vi "NumericPad-DM.vi"(0 "Input Cluster":T2={"Operation"=0, "Wait for (ms):"=1000, "Look for key press:"=49} {"Look for key press:" items=["Key_1"=49, "Key_2"=50, "Key_3"=51, "Key_4"=52, "Key_5"=53, "Key_6"=54, "Key_7"=55, "Key_8"=56, "Key_9"=57, "Key_0"=48, "Key_#"=35, "Key_*"=42]; "Operation" items=["ReadPad", "InitializeSetup"]}, 2 "NXT":T3={"error"={"status"=FALSE, "code"=0, "source"=""}, "address"="USB0::0x0694::0x0002::001653FF017B::RAW", "NXT #"=0, "Show Error"=TRUE, "Connection"=4} {"Connection" items=["USB", "Bluetooth", "USB then Bluetooth", "Last Connection", "Preference"]}, 3 "Input Port":T4 items=["Port 1", "Port 2", "Port 3", "Port 4"]) -> (1 "Output Cluster":T1={"Key Numeric Value"=49, "Key String Value"="1", "Key match found"=FALSE}, 4 "NXT dup":T3={"error"={"status"=FALSE, "code"=0, "source"=""}, "address"="USB0::0x0694::0x0002::001653FF017B::RAW", "NXT #"=0, "Show Error"=TRUE, "Connection"=4} {"Connection" items=["USB", "Bluetooth", "USB then Bluetooth", "Last Connection", "Preference"]})   [LabVIEW 2009]
uses:
  <vilib>/NXT/Subs/LVHSConnector.ctl
  <vilib>/NXT/Block Support/NXT_InputPort.ctl
  <vilib>/NXT/Block Support/HWPage.SensorType.ctl
  <vilib>/NXT/Block Support/HWPage.SensorMode.ctl
  <vilib>/NXT/Dual Mode Library/Waits/Wait_Num(msec).vi
panel:
  out "Look for key press:":u8(ring)=49 caption="Operation" items=["Key_1"=49, "Key_2"=50, "Key_3"=51, "Key_4"=52, "Key_5"=53, "Key_6"=54, "Key_7"=55, "Key_8"=56, "Key_9"=57, "Key_0"=48, "Key_#"=35, "Key_*"=42]
  out "Key match found":bool
  in  "keymapS":string[](array[string])=[" ", " ", " ", " ", "4", "1", "7", "*", "5", "2", "8", "0", "3", "6", "9", "#"]
  out "Key String Value":string="1"
  in  "keyMapN":u8[](array[numeric])=[0, 0, 0, 0, 52, 49, 55, 42, 53, 50, 56, 48, 51, 54, 57, 35, 119] format="%x"
  out "Key Numeric Value":u8=49
  out "KeyPos":u8=5 format="%x"
  # "mindsensors.com\nCopyright (c) 2009 by mindsensors.com\nEmail: info (<at>) mindsensors (<dot>) com\n\nThis program is free software. You can redistribute it and/or modify\nit under the terms of the GNU General Public License as published by\nthe Free Software Foundation; version 3 of the License.\nRead the license at: http://www.gnu.org/licenses/gpl.txt"
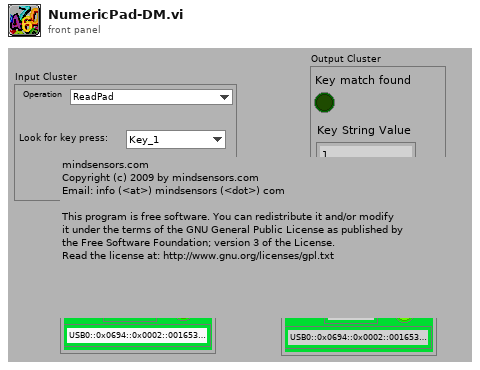
[diagram p1: front panel]
types:
  T1 = cluster{"Key Numeric Value":u8, "Key String Value":string, "Key match found":bool}
  T2 = cluster{"Operation":u8, "Wait for (ms):":i16, "Look for key press:":u8}
  T3 = typedef "LVHSConnector.ctl" = cluster{"error":errorcluster, "address":string, "NXT #":i32, "Show Error":bool, "Connection":u16}
  T4 = typedef "NXT_InputPort.ctl" = u8
  T5 = typedef "HWPage.SensorType.ctl" = u8
  T6 = typedef "HWPage.SensorMode.ctl" = u8
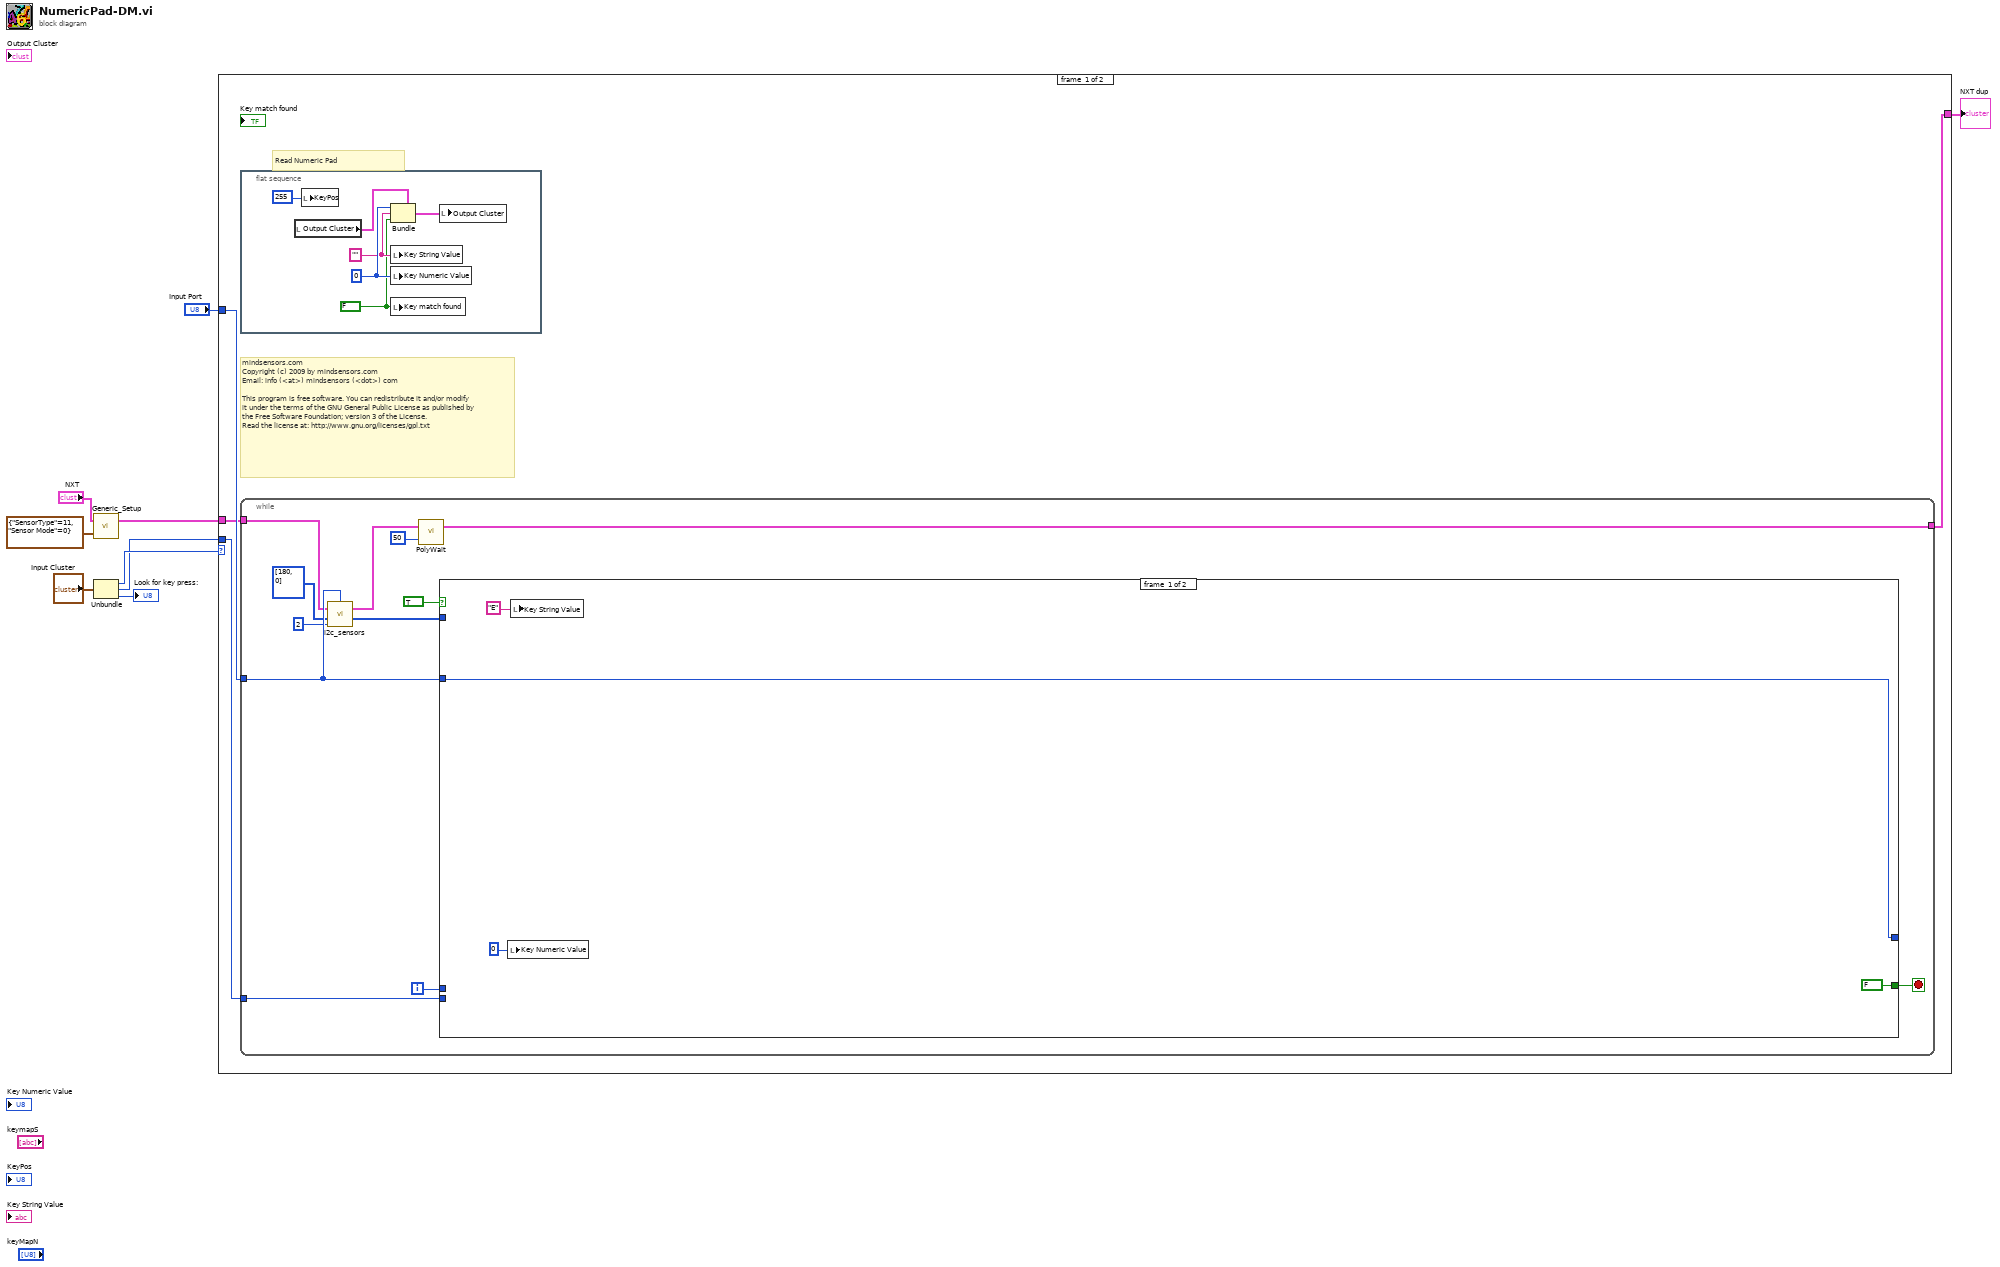
[diagram p0: block diagram]
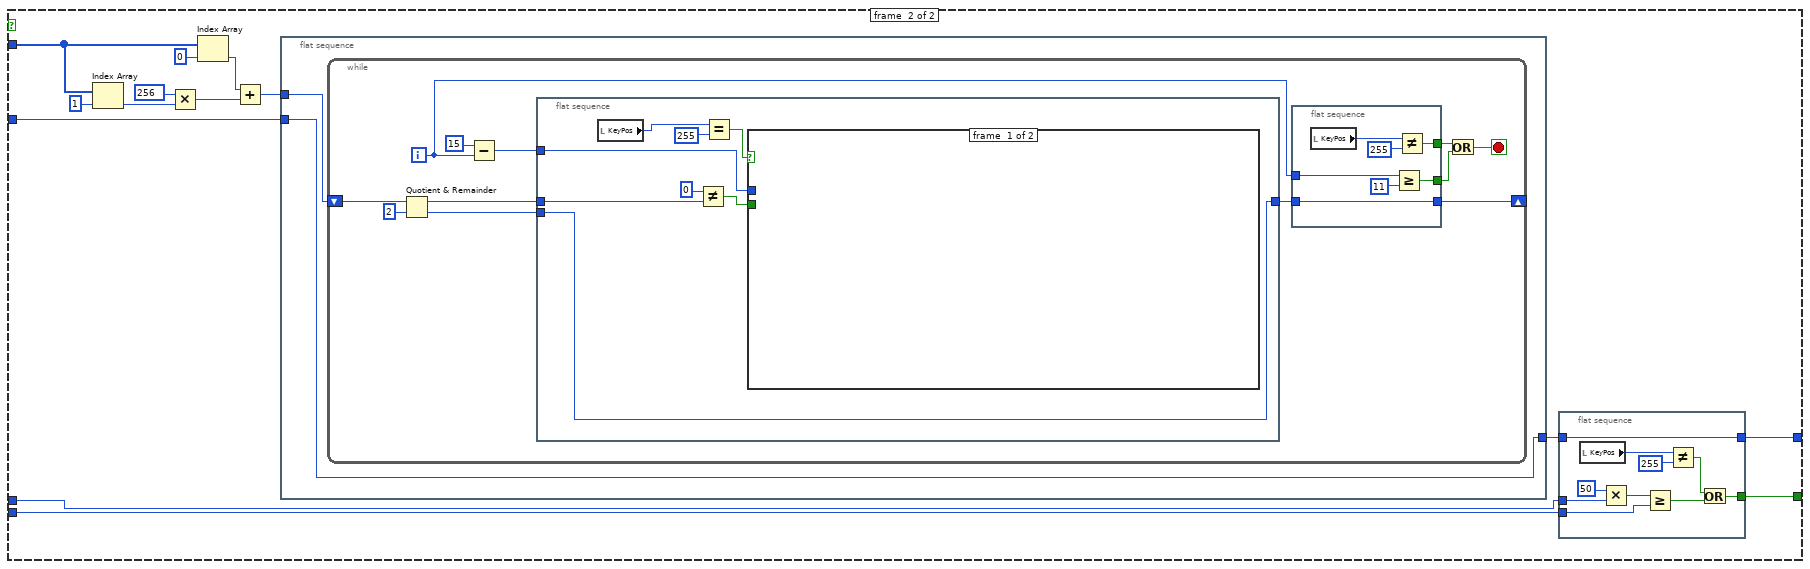
[diagram p2: hidden frame]
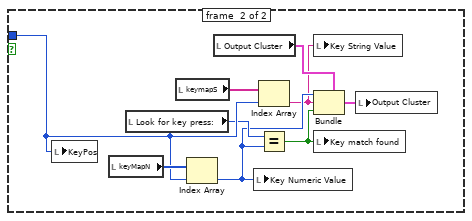
[diagram p4: hidden frame]
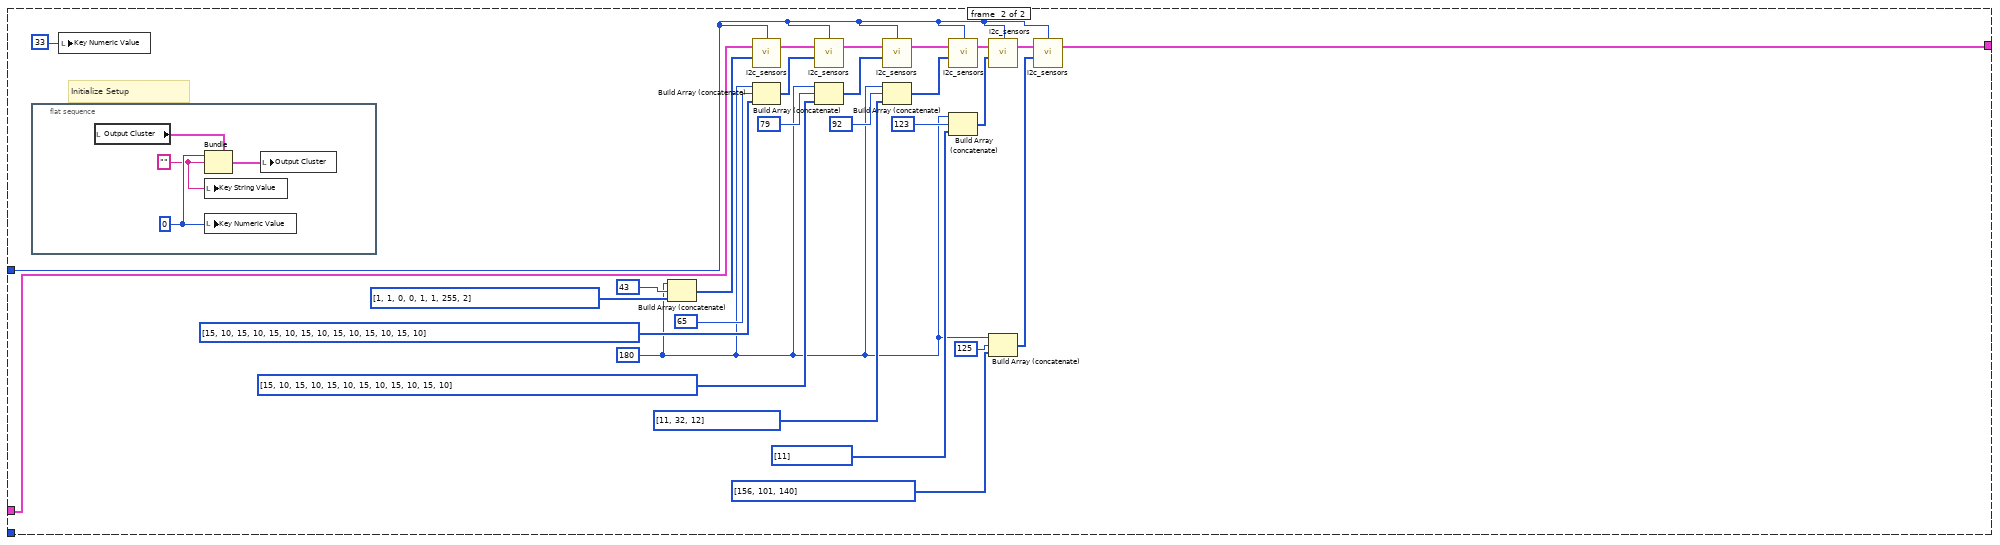
[diagram p5: hidden frame]
diagram:
  n1 = call <vilib>:"Generic_Setup.vi"("Sensor Setup"=cluster{"SensorType":T5, "Sensor Mode":T6} {"SensorType"=11, "Sensor Mode"=0}, "NXT"="NXT") -> ("NXT"=w6:T3)  [unwired: 1 in, 1 out]
  n2 = Unbundle("Input Cluster") -> ("Operation"=w3:u8, "Wait for (ms):"=w2:i16, "Look for key press:"=→"Look for key press:":u8)
  n3 = case shown="0" w3 {
    tunnel: w2 -> [w13 _]
    tunnel: "Input Port" -> [w12 w102]
    tunnel: w6 -> [w11 w123]
    tunnel: [w10 w101] -> w5
    frame #0 {
      # "mindsensors.com\nCopyright (c) 2009 by mindsensors.com\nEmail: info (<at>) mindsensors (<dot>) com\n\nThis program is free software. You can redistribute it and/or modify\nit under the terms of the GNU General Public License as published by\nthe Free Software Foundation; version 3 of the License.\nRead the license at: http://www.gnu.org/licenses/gpl.txt"
      # "Read Numeric Pad"
      n4 = flat-sequence {
        frame #0 {
          w14 = FALSE ("keyMatched")
          w16 = u8 0 ("keyN")
          w15 = "" ("keyS")
          n5 = local read "Output Cluster"() -> (w18:T1)
          n6 = local write "KeyPos"(u8 255 ("Key Value")) -> ()
          n7 = Bundle(cluster=w18, "Key Numeric Value"=w16, "Key String Value"=w15, "Key match found"=w14) -> (w17:T1)
          n8 = local write "Key String Value"(w15) -> ()
          n9 = local write "Key Numeric Value"(w16) -> ()
          n10 = local write "Key match found"(w14) -> ()
          n11 = local write "Output Cluster"(w17) -> ()
        }
      }
      n12 = while {
        tunnel: w13 -> [w29]
        tunnel: w12 -> [w28]
        tunnel: w11 -> [w26]
        tunnel: [w23] -> w10
        i -> [w30]
        stop <- w31 stop-if-true
        n13 = call <vilib>:"i2c_sensors.vi"("Return Length"=u8 2, "Bytes to Write"=u8[] [180, 0] ("Buffer"), "NXT"=w26, "Port"=w28) -> ("Bytes read"=w27:u8[], "NXT"=w24:T3)  [unwired: 1 in, 1 out]
        n14 = call-poly <vilib>:"PolyWait.vi"("Time (100 msec)"=u16 50 ("Delay ms"), "NXT"=w24) -> ("NXT"=w23:T3)  [unwired: 2 in]
        n15 = case shown="True" TRUE {
          tunnel: w27 -> [_ w44]
          tunnel: [FALSE w37] -> w31
          tunnel: w28 -> [w35 w42]
          tunnel: [w35 w40] -> _
          tunnel: w30 -> [_ w39]
          tunnel: w29 -> [_ w38]
          frame #0 {
            n16 = local write "Key Numeric Value"(u8 0 ("keyN")) -> ()
            n17 = local write "Key String Value"("E" ("keyS")) -> ()
          }
          frame #1 {
            n18 = Index Array(array=w44, index=1) -> (element=w48:u8)
            n19 = Multiply(x=u16 256, y=w48) -> (x*y=w46:u16)
            n20 = Index Array(array=w44, index=0) -> (element=w47:u8)
            n21 = Add(x=w47, y=w46) -> (x+y=w43:u16)
            n22 = flat-sequence {
              tunnel: w43 -> [w61]
              tunnel: w42 -> [w60]
              tunnel: [w60] -> w41
              frame #0 {
                n23 = while {
                  shift-right: [w69] -> _
                  shift-left: w61 -> [w72]
                  i -> [w64]
                  stop <- w67 stop-if-true
                  n24 = Quotient & Remainder(x=w72, y=u8 2) -> (x-y*floor(x/y)=w68:u16, floor(x/y)=w71:u16)
                  n25 = Subtract(x=15, y=w64) -> (x-y=w65:i32)
                  n26 = flat-sequence {
                    tunnel: w71 -> [w88]
                    tunnel: [w88] -> w70
                    tunnel: w68 -> [w86]
                    tunnel: w65 -> [w85]
                    frame #0 {
                      n27 = local read "KeyPos"() -> (w83:u8)
                      n28 = Not Equal?(x=u16 0, y=w86) -> (x != y?=w87:bool)
                      n29 = Equal?(x=w83, y=u8 255 ("Key Value")) -> (x = y?=w82:bool)
                      n30 = case shown="True" w82 {
                        tunnel: w87 -> [_ w90]
                        tunnel: w85 -> [_ w89]
                        frame #0 {
                        }
                        frame #1 {
                          n31 = case shown="True" w90 {
                            tunnel: w89 -> [_ w97]
                            frame #0 {
                            }
                            frame #1 {
                              n32 = local write "KeyPos"(w97) -> ()
                              n33 = local read "keyMapN"() -> (w99:u8[])
                              n34 = local read "Look for key press:"() -> (w96:u8)
                              n35 = local read "keymapS"() -> (w98:string[])
                              n36 = Index Array(array=w99, index=w97) -> (element=w92:u8)
                              n37 = local read "Output Cluster"() -> (w94:T1)
                              n38 = local write "Key Numeric Value"(w92) -> ()
                              n39 = Index Array(array=w98, index=w97) -> (element=w91:string)
                              n40 = Equal?(x=w96, y=w92) -> (x = y?=w93:bool)
                              n41 = local write "Key String Value"(w91) -> ()
                              n42 = Bundle(cluster=w94, "Key Numeric Value"=w92, "Key String Value"=w91, "Key match found"=w93) -> (w95:T1)
                              n43 = local write "Key match found"(w93) -> ()
                              n44 = local write "Output Cluster"(w95) -> ()
                            }
                          }
                        }
                      }
                    }
                  }
                  n45 = flat-sequence {
                    tunnel: w70 -> [w80]
                    tunnel: [w80] -> w69
                    tunnel: [w78] -> w62
                    tunnel: w64 -> [w76]
                    tunnel: [w75] -> w66
                    frame #0 {
                      n46 = local read "KeyPos"() -> (w79:u8)
                      n47 = Greater Or Equal?(x=w76, y=u8 11) -> (x >= y?=w75:bool)
                      n48 = Not Equal?(x=w79, y=u8 255 ("Key Value")) -> (x != y?=w78:bool)
                    }
                  }
                  n49 = Or(x=w62, y=w66) -> (x .or. y?=w67:bool)
                }
              }
            }
            n50 = flat-sequence {
              tunnel: w41 -> [w59]
              tunnel: [w59] -> w40
              tunnel: w39 -> [w58]
              tunnel: w38 -> [w56]
              tunnel: [w57] -> w37
              frame #0 {
                n51 = local read "KeyPos"() -> (w52:u8)
                n52 = Multiply(x=50, y=w58) -> (x*y=w54:i32)
                n53 = Greater Or Equal?(x=w54, y=w56) -> (x >= y?=w53:bool)
                n54 = Not Equal?(x=w52, y=u8 255 ("Key Value")) -> (x != y?=w51:bool)
                n55 = Or(x=w51, y=w53) -> (x .or. y?=w57:bool)
              }
            }
          }
        }
      }
    }
    frame #1 {
      w100 = u8 180
      # "Initialize Setup"
      n56 = flat-sequence {
        frame #0 {
          w129 = u8 0 ("keyN")
          w128 = "" ("keyS")
          n57 = local read "Output Cluster"() -> (w131:T1)
          n58 = Bundle(cluster=w131, "Key Numeric Value"=w129, "Key String Value"=w128) -> (w130:T1)  [unwired: 1 in]
          n59 = local write "Key String Value"(w128) -> ()
          n60 = local write "Key Numeric Value"(w129) -> ()
          n61 = local write "Output Cluster"(w130) -> ()
        }
      }
      n62 = local write "Key Numeric Value"(u8 33 ("keyN")) -> ()
      n63 = Build Array (concatenate)(w100, 43, u8[] [1, 1, 0, 0, 1, 1, 255, 2]) -> (w124:i32[])
      n64 = call <vilib>:"i2c_sensors.vi"("Bytes to Write"=w124, "NXT"=w123, "Port"=w102) -> ("NXT"=w103:T3)  [unwired: 2 in, 2 out]
      n65 = Build Array (concatenate)(w100, 65, u8[] [15, 10, 15, 10, 15, 10, 15, 10, 15, 10, 15, 10, 15, 10]) -> (w112:i32[])
      n66 = call <vilib>:"i2c_sensors.vi"("Bytes to Write"=w112, "NXT"=w103, "Port"=w102) -> ("NXT"=w104:T3)  [unwired: 2 in, 2 out]
      n67 = Build Array (concatenate)(w100, 79, u8[] [15, 10, 15, 10, 15, 10, 15, 10, 15, 10, 15, 10]) -> (w111:i32[])
      n68 = call <vilib>:"i2c_sensors.vi"("Bytes to Write"=w111, "NXT"=w104, "Port"=w102) -> ("NXT"=w105:T3)  [unwired: 2 in, 2 out]
      n69 = Build Array (concatenate)(w100, 92, i32[] [11, 32, 12]) -> (w110:i32[])
      n70 = call <vilib>:"i2c_sensors.vi"("Bytes to Write"=w110, "NXT"=w105, "Port"=w102) -> ("NXT"=w106:T3)  [unwired: 2 in, 2 out]
      n71 = Build Array (concatenate)(w100, 123, i32[] [11]) -> (w109:i32[])
      n72 = call <vilib>:"i2c_sensors.vi"("Bytes to Write"=w109, "NXT"=w106, "Port"=w102) -> ("NXT"=w107:T3)  [unwired: 2 in, 2 out]
      n73 = Build Array (concatenate)(w100, 125, u8[] [156, 101, 140]) -> (w108:i32[])
      n74 = call <vilib>:"i2c_sensors.vi"("Bytes to Write"=w108, "NXT"=w107, "Port"=w102) -> ("NXT"=w101:T3)  [unwired: 2 in, 2 out]
    }
  }
  "NXT dup" <- w5
